vi "GetPlots.vi"(8 "error in":errorcluster, 11 "WaveformChart in":refnum<class "WaveformGraph.lvclass">) -> (0 "error out":errorcluster, 3 "WaveformChart out":refnum<class "WaveformGraph.lvclass">)   [LabVIEW 2014, in "WaveformGraph.lvclass"]
uses:
  WaveformGraph.lvclass
  WaveformGraph.lvclass/WaveformGraph.ctl
  Plot/Plot.lvclass
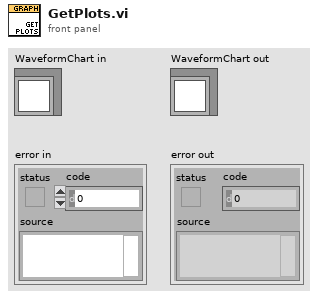
[diagram p1: front panel]
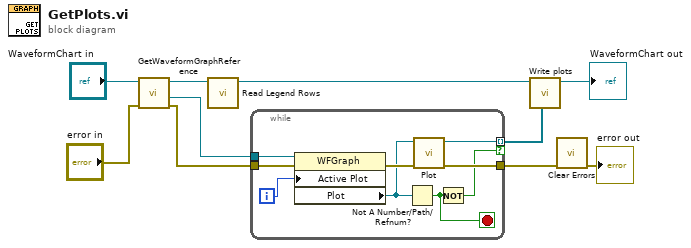
[diagram p0: block diagram]
diagram:
  n1 = call "GetWaveformGraphReference.vi"("error in"="error in", "WFGraph in"="WaveformChart in") -> ("error out"=w10:errorcluster, "WFGraph reference"=w9:refnum<vi>, "WFGraph out"=w7:refnum<class "WaveformGraph.lvclass">)  [unwired: 7 in]
  n2 = call "Read Legend Rows.vi"("WaveformChart in"=w7) -> ("WaveformChart out"=w5:refnum<class "WaveformGraph.lvclass">)  [unwired: 7 in, 1 out]
  n3 = while {
    tunnel: w9 -> [w18]
    tunnel: [w14] -> w8 mode=indexing if=w12
    tunnel: w10 -> [w19]
    tunnel: [w15] -> w3
    i -> [w17]
    stop <- w11 stop-if-true
    n4 = property class="WFGraph"(reference=w18, error in=w19, "Active Plot"=w17) -> (error out=w16:errorcluster, "Plot"=w13:refnum<vi>)  [unwired: 1 out]
    n5 = Not A Number/Path/Refnum?(number/path/refnum=w13) -> (NaN/Path/Refnum?=w11:bool)
    n6 = call "Plot.vi"("error in"=w16, "Plot Refnum"=w13) -> ("error out"=w15:errorcluster, "Plot out"=w14:refnum<class "Plot.lvclass">)  [unwired: 8 in]
    n7 = Not(x=w11) -> (.not. x?=w12:bool)
  }
  n8 = call "Write plots.vi"("plots"=w8, "WaveformGraph in"=w5) -> ("WaveformGraph out"=→"WaveformChart out":refnum<class "WaveformGraph.lvclass">)  [unwired: 7 in]
  n9 = call <vilib>:"Clear Errors.vi"("error in (no error)"=w3) -> ("error out"=→"error out":errorcluster)  [unwired: 5 in, 1 out]
